vi "Set Fields.vi"(8 "error in":errorcluster, 10 "Fields Cluster":variant, 11 "Device Info in":refnum<class "Device Info.lvclass">) -> (0 "error out":errorcluster, 3 "Device Info out":refnum<class "Device Info.lvclass">)   [LabVIEW 2024, in "EDS.lvlib" / "Device Info.lvclass"]
uses:
  Device Info.lvclass
  Device Info.lvclass/Device Info.ctl
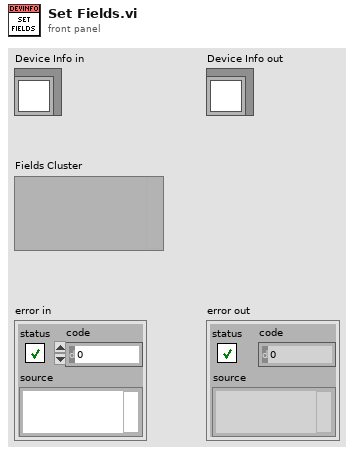
[diagram p1: front panel]
types:
  T1 = cluster{"ProductName":string, "ProductNumber":string, "VendorName":string, "VendorNumber":string, "RevisionNumber":string, "OrderCode":string, "BaudRate_10":bool, "BaudRate_20":bool, "BaudRate_50":bool, "BaudRate_125":bool, "BaudRate_250":bool, "BaudRate_500":bool, "BaudRate_800":bool, "BaudRate_1000":bool, "SimpleBootUpMaster":bool, "SimpleBootUpSlave":bool, "Granularity":i16, "DynamicChannelsSupported":bool, "CompactPDO":bool, "GroupMessaging":bool, "NrOfRXPDO":i16, "NrOfTXPDO":i16, "LSS_Supported":bool}
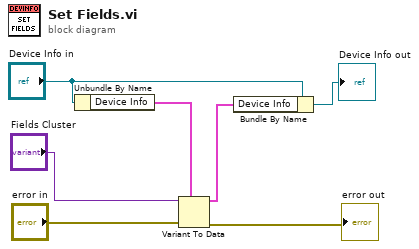
[diagram p0: block diagram]
diagram:
  n1 = Unbundle By Name("Device Info in") -> ("Device Info"=w5:T1)
  n2 = Variant To Data(error in="error in", type=w5, Variant="Fields Cluster") -> (data=w1:T1, error out=→"error out":errorcluster)
  n3 = Bundle By Name(cluster="Device Info in", "Device Info"=w1) -> (→"Device Info out":refnum<class "Device Info.lvclass">)
